vi "BundleCompareBits.vi"(5 "Expected Value(s)":u8[](array[numeric]), 7 "Compare Locations":u32[](array[numeric]), 11 "Compare Bits In":T1[](array[typedef]) {"Expected Value(s)" format="%.0x"}) -> (3 "Compare Bits Out":T1[](array[typedef]) {"Expected Value(s)" format="%.0x"})   [LabVIEW 2013]
doc: "Bundles expected value(s) and compare locations for the process data VI. This VI is only needed when reading data when the expected value is unknown or to detect parity errors."
uses:
  Ctrls/ReadInfo.ctl
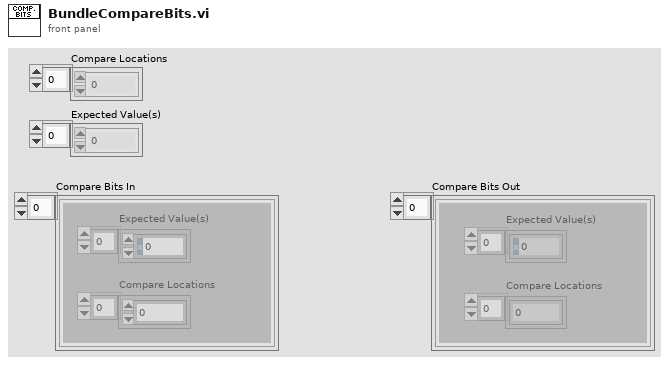
[diagram p1: front panel]
types:
  T1 = typedef "ReadInfo.ctl" = cluster{"Expected Value(s)":u8[], "Compare Locations":u32[]}
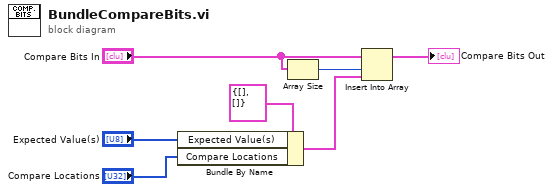
[diagram p0: block diagram]
diagram:
  n1 = Bundle By Name(cluster=T1 {"Expected Value(s)"=[], "Compare Locations"=[]} ("Read Info"), "Expected Value(s)"="Expected Value(s)", "Compare Locations"="Compare Locations") -> (w7:T1)
  n2 = Array Size(array="Compare Bits In") -> (size(s)=w6:i32)
  n3 = Insert Into Array(array="Compare Bits In", index=w6, new element=w7) -> (→"Compare Bits Out":T1[])
